vi "IrrevantSubTree.vi"(0 "best dist":dbl, 1 "Bounding Box":dbl[](array[numeric]), 2 "target":dbl[](array[numeric])) -> (8 "Irrelevant subTree":bool)   [LabVIEW 2016]
uses:
  <vilib>/Analysis/_algsub.llb/Real Vector Norm.vi
  <vilib>/Analysis/NI_AALPro.lvlib
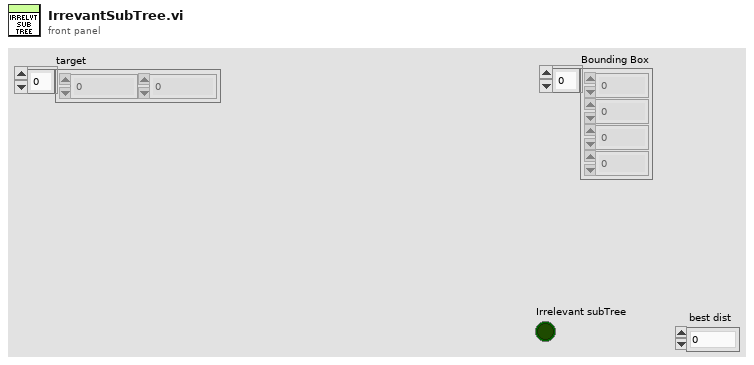
[diagram p1: front panel]
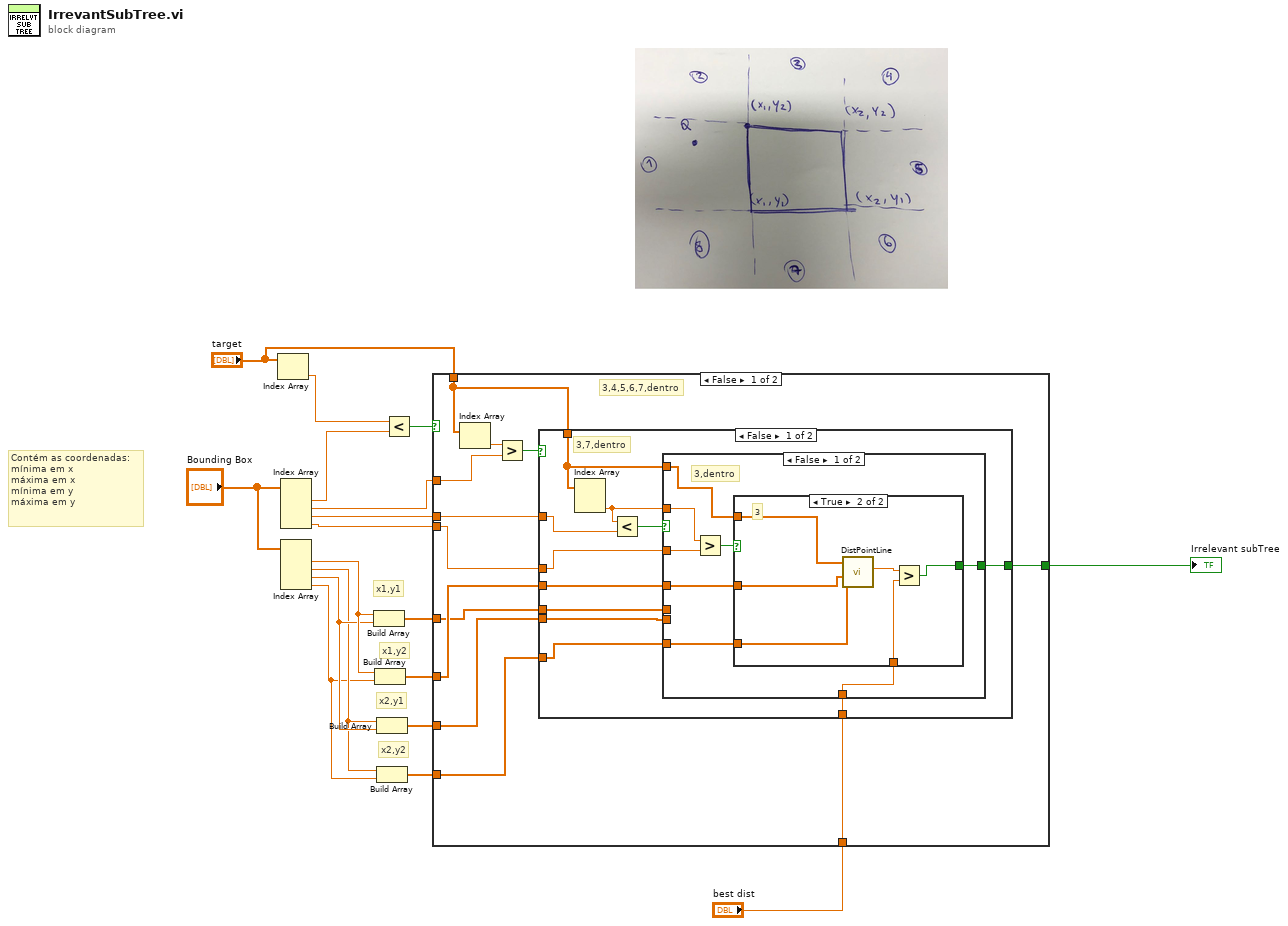
[diagram p0: block diagram]
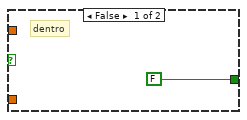
[diagram p2: hidden frame]
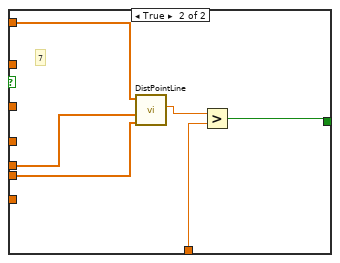
[diagram p3: hidden frame]
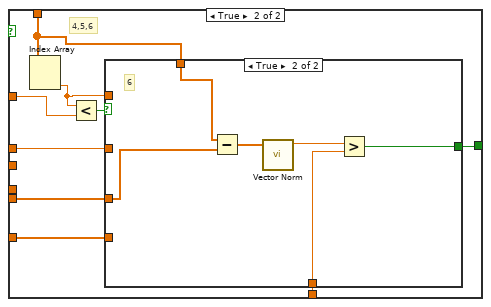
[diagram p4: hidden frame]
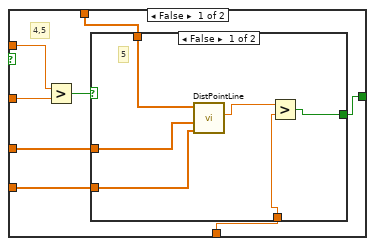
[diagram p5: hidden frame]
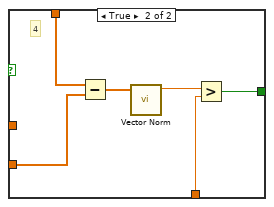
[diagram p6: hidden frame]
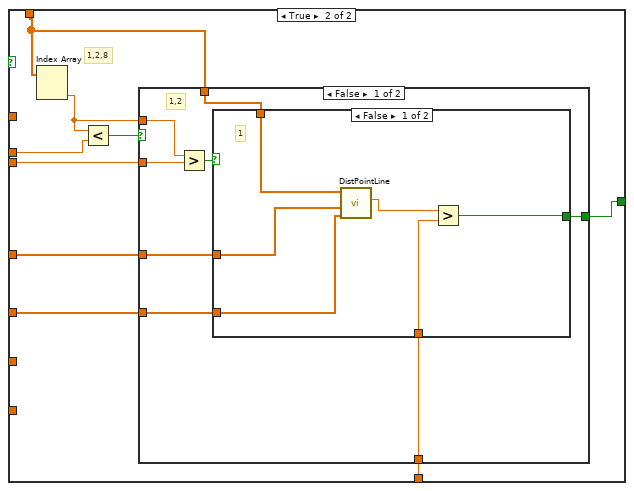
[diagram p7: hidden frame]
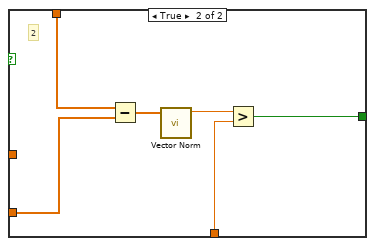
[diagram p8: hidden frame]
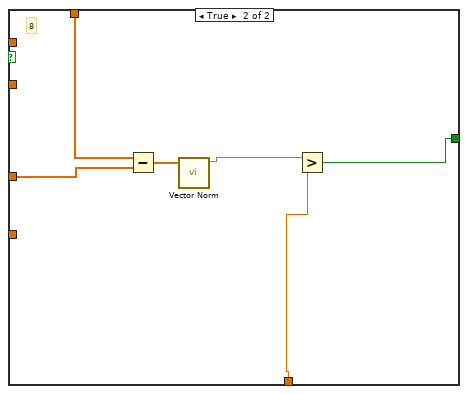
[diagram p9: hidden frame]
diagram:
  # "x2,y2"
  # "x2,y1"
  # "x1,y2"
  # "x1,y1"
  # "Contém as coordenadas:\nmínima em x\nmáxima em x\nmínima em y\nmáxima em y"
  n1 = Index Array(array="target") -> (element=w16:dbl)  [unwired: 1 in]
  n2 = Index Array(array="Bounding Box") -> (element #1=w17:dbl, element #2=w12:dbl, element #3=w14:dbl, element #4=w13:dbl)  [unwired: 4 in]
  n3 = Index Array(array="Bounding Box") -> (element #1=w9:dbl, element #2=w7:dbl, element #3=w8:dbl, element #4=w6:dbl)  [unwired: 4 in]
  n4 = Build Array(w9, w8) -> (w5:dbl[])
  n5 = Build Array(w9, w6) -> (w4:dbl[])
  n6 = Build Array(w7, w8) -> (w3:dbl[])
  n7 = Build Array(w7, w6) -> (w2:dbl[])
  n8 = Less?(x=w16, y=w17) -> (x < y?=w18:bool)
  n9 = case shown="False" w18 {
    tunnel: "target" -> [w27 w102]
    tunnel: w14 -> [w26 w105]
    tunnel: w13 -> [w25 w103]
    tunnel: w12 -> [w29 _]
    tunnel: [w24 w98] -> w11
    tunnel: w5 -> [w20 w101]
    tunnel: w4 -> [w22 w100]
    tunnel: w3 -> [w23 _]
    tunnel: w2 -> [w21 _]
    tunnel: "best dist" -> [w19 w99]
    frame False {
      # "3,4,5,6,7,dentro"
      n10 = Index Array(array=w27) -> (element=w30:dbl)  [unwired: 1 in]
      n11 = Greater?(x=w30, y=w29) -> (0:w28:bool)
      n12 = case shown="False" w28 {
        tunnel: w27 -> [w32 w65]
        tunnel: w26 -> [w40 w70]
        tunnel: w25 -> [w38 w68]
        tunnel: [w37 w63] -> w24
        tunnel: w23 -> [w33 w67]
        tunnel: w21 -> [w35 w66]
        tunnel: w22 -> [w36 _]
        tunnel: w20 -> [w34 _]
        tunnel: w19 -> [w31 w64]
        frame False {
          # "3,7,dentro"
          n13 = Index Array(array=w32) -> (element #2=w39:dbl)  [unwired: 2 in, 1 out]
          n14 = Less?(x=w39, y=w40) -> (x < y?=w41:bool)
          n15 = case shown="False" w41 {
            tunnel: w39 -> [w48 _]
            tunnel: w38 -> [w47 _]
            tunnel: [w46 w57] -> w37
            tunnel: w36 -> [w45 _]
            tunnel: w35 -> [w44 _]
            tunnel: w34 -> [_ w61]
            tunnel: w33 -> [_ w60]
            tunnel: w32 -> [w43 w62]
            tunnel: w31 -> [w42 w58]
            frame False {
              # "3,dentro"
              n16 = Greater?(x=w48, y=w47) -> (0:w49:bool)
              n17 = case shown="True" w49 {
                tunnel: [FALSE w51] -> w46
                tunnel: w45 -> [_ w55]
                tunnel: w44 -> [_ w54]
                tunnel: w43 -> [_ w56]
                tunnel: w42 -> [_ w52]
                frame False {
                  # "dentro"
                }
                frame True {
                  # "3"
                  n18 = call "DistPointLine.vi"("P2"=w54, "P1"=w55, "Q"=w56) -> ("distance"=w53:dbl)  [unwired: 8 in]
                  n19 = Greater?(x=w53, y=w52) -> (0:w51:bool)
                }
              }
            }
            frame True {
              # "7"
              n20 = call "DistPointLine.vi"("P2"=w60, "P1"=w61, "Q"=w62) -> ("distance"=w59:dbl)  [unwired: 8 in]
              n21 = Greater?(x=w59, y=w58) -> (0:w57:bool)
            }
          }
        }
        frame True {
          # "4,5,6"
          n22 = Index Array(array=w65) -> (element #2=w69:dbl)  [unwired: 2 in, 1 out]
          n23 = Less?(x=w69, y=w70) -> (x < y?=w71:bool)
          n24 = case shown="True" w71 {
            tunnel: w69 -> [w78 _]
            tunnel: w68 -> [w77 _]
            tunnel: w67 -> [w76 w95]
            tunnel: w66 -> [w75 _]
            tunnel: w65 -> [w74 w96]
            tunnel: w64 -> [w73 w93]
            tunnel: [w72 w92] -> w63
            frame False {
              # "4,5"
              n25 = Greater?(x=w78, y=w77) -> (0:w79:bool)
              n26 = case shown="False" w79 {
                tunnel: w76 -> [w84 _]
                tunnel: w75 -> [w83 w89]
                tunnel: w74 -> [w85 w90]
                tunnel: w73 -> [w81 w87]
                tunnel: [w80 w86] -> w72
                frame False {
                  # "5"
                  n27 = call "DistPointLine.vi"("P2"=w83, "P1"=w84, "Q"=w85) -> ("distance"=w82:dbl)  [unwired: 8 in]
                  n28 = Greater?(x=w82, y=w81) -> (0:w80:bool)
                }
                frame True {
                  # "4"
                  n29 = Subtract(x=w90, y=w89) -> (x-y=w91:dbl[])
                  n30 = call-poly <vilib>:"Vector Norm.vi"("Input Vector"=w91) -> ("norm"=w88:dbl)  [unwired: 9 in, 1 out]
                  n31 = Greater?(x=w88, y=w87) -> (0:w86:bool)
                }
              }
            }
            frame True {
              # "6"
              n32 = Subtract(x=w96, y=w95) -> (x-y=w97:dbl[])
              n33 = call-poly <vilib>:"Vector Norm.vi"("Input Vector"=w97) -> ("norm"=w94:dbl)  [unwired: 9 in, 1 out]
              n34 = Greater?(x=w94, y=w93) -> (0:w92:bool)
            }
          }
        }
      }
    }
    frame True {
      # "1,2,8"
      n35 = Index Array(array=w102) -> (element #2=w104:dbl)  [unwired: 2 in, 1 out]
      n36 = Less?(x=w104, y=w105) -> (x < y?=w106:bool)
      n37 = case shown="False" w106 {
        tunnel: w104 -> [w114 _]
        tunnel: w103 -> [w112 _]
        tunnel: w102 -> [w109 w131]
        tunnel: w101 -> [w110 w130]
        tunnel: w100 -> [w111 _]
        tunnel: w99 -> [w108 w128]
        tunnel: [w107 w127] -> w98
        frame False {
          # "1,2"
          n38 = Greater?(x=w114, y=w112) -> (0:w113:bool)
          n39 = case shown="False" w113 {
            tunnel: w111 -> [w118 w124]
            tunnel: w110 -> [w119 _]
            tunnel: w109 -> [w120 w125]
            tunnel: w108 -> [w116 w122]
            tunnel: [w115 w121] -> w107
            frame False {
              # "1"
              n40 = call "DistPointLine.vi"("P2"=w118, "P1"=w119, "Q"=w120) -> ("distance"=w117:dbl)  [unwired: 8 in]
              n41 = Greater?(x=w117, y=w116) -> (0:w115:bool)
            }
            frame True {
              # "2"
              n42 = Subtract(x=w125, y=w124) -> (x-y=w126:dbl[])
              n43 = call-poly <vilib>:"Vector Norm.vi"("Input Vector"=w126) -> ("norm"=w123:dbl)  [unwired: 9 in, 1 out]
              n44 = Greater?(x=w123, y=w122) -> (0:w121:bool)
            }
          }
        }
        frame True {
          # "8"
          n45 = Subtract(x=w131, y=w130) -> (x-y=w132:dbl[])
          n46 = call-poly <vilib>:"Vector Norm.vi"("Input Vector"=w132) -> ("norm"=w129:dbl)  [unwired: 9 in, 1 out]
          n47 = Greater?(x=w129, y=w128) -> (0:w127:bool)
        }
      }
    }
  }
  "Irrelevant subTree" <- w11
